vi "Configure Current Limit.vi"(8 "error in (no error)":errorcluster, 10 "Set Current":dbl format="%.1g", 11 "VISA resource name":refnum<visa-resource-name>) -> (0 "error out":errorcluster, 3 "VISA resource name out":refnum<visa-resource-name>)   [LabVIEW 2021, in "BK Precision 169XB.lvlib"]
doc: "Configures over current protection (OCP). Specify the output current limit value and the behavior of the power supply when the output current is greater than or equal to that value."
uses:
  BK Precision 169XB.lvlib
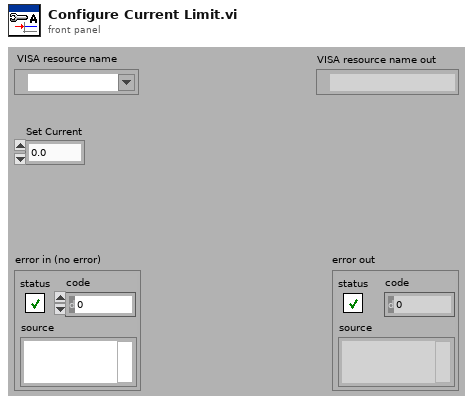
[diagram p1: front panel]
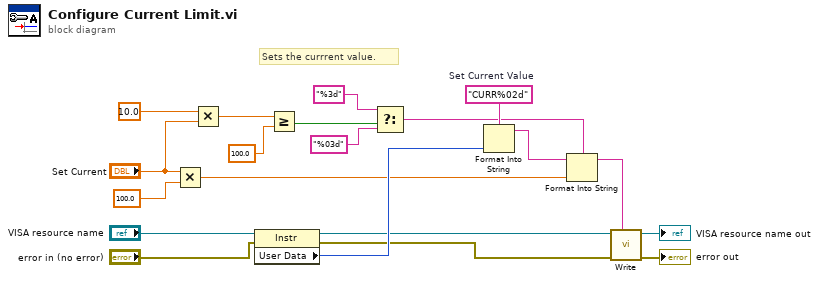
[diagram p0: block diagram]
diagram:
  w10 = "CURR%02d"  # Set Current Value
  # "Sets the currrent value."
  n1 = Multiply(x="Set Current", y=100.0) -> (x*y=w3:dbl)
  n2 = Multiply(x="Set Current", y=10.0) -> (x*y=w18:dbl)
  n3 = property class="Instr"(reference="VISA resource name", error in="error in (no error)") -> (reference out=w7:refnum<visa-resource-name>, error out=w6:errorcluster, "User Data"=w9:u32)
  n4 = Greater Or Equal?(x=w18, y=100.0) -> (x >= y?=w16:bool)
  n5 = Select(t="%3d" ("format string"), s=w16, f="%03d" ("format string")) -> (s? t:f=w4:string)
  n6 = Format Into String(format string=w10, w9) -> (resulting string=w2:string)  [unwired: 2 in, 1 out]
  n7 = Format Into String(format string=w4, initial string=w2, w3) -> (resulting string=w1:string)  [unwired: 1 in, 1 out]
  n8 = call "Write.vi"("Input String"=w1, "error in (no error)"=w6, "VISA resource name"=w7) -> ("error out"=→"error out":errorcluster, "VISA resource name out"=→"VISA resource name out":refnum<visa-resource-name>)  [unwired: 6 in, 1 out]
